vi "Test - Read Tuner Type.vi"() -> ()   [LabVIEW 2020]
uses:
  RTL-SDR/Device/Device.lvclass
  RTL-SDR/Session/Session.lvclass
  RTL-SDR/Tuner Type.ctl
  RTL-SDR/RTL-SDR.lvlib
panel:
  out "Tuner Gains":dbl[](array[numeric])
  out "error out":errorcluster
  out "Tuner Type":T1
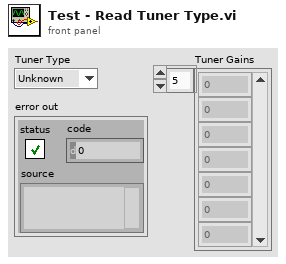
[diagram p1: front panel]
types:
  T1 = typedef "RTL-SDR.lvlib/Tuner Type.ctl" = enum32{"Unknown", "E4000", "FC0012", "FC0013", "FC2580", "R820T", "R828D"}
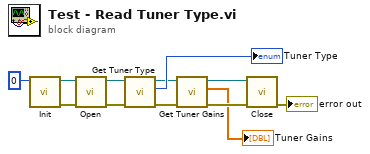
[diagram p0: block diagram]
diagram:
  n1 = call "Init.vi"("Index"=0) -> ("error out"=w10:errorcluster, "Device out"=w11:refnum<class "Device.lvclass">)  [unwired: 9 in]
  n2 = call "Open.vi"("error in (no error)"=w10, "Device"=w11) -> ("error out"=w8:errorcluster, "RTL-SDR out"=w9:refnum<class "Session.lvclass">)  [unwired: 8 in]
  n3 = call "Get Tuner Type.vi"("error in (no error)"=w8, "RTL-SDR in"=w9) -> ("error out"=w4:errorcluster, "Tuner Type"=→"Tuner Type":T1, "RTL-SDR out"=w5:refnum<class "Session.lvclass">)  [unwired: 7 in]
  n4 = call "Get Tuner Gains.vi"("error in (no error)"=w4, "RTL-SDR in"=w5) -> ("error out"=w2:errorcluster, "Tuner Gains"=→"Tuner Gains":dbl[], "RTL-SDR out"=w3:refnum<class "Session.lvclass">)  [unwired: 7 in]
  n5 = call "Close.vi"("error in (no error)"=w2, "RTL-SDR in"=w3) -> ("error out"=→"error out":errorcluster)  [unwired: 8 in, 1 out]
